vi "ModbusRead.vi"() -> ()   [LabVIEW 2023]
uses:
  <vilib>/NI/Modbus Library/API/Wrapper/Create TCP Master.vi
  <vilib>/NI/Modbus Library/API/Master/Modbus Master.lvclass
  <vilib>/NI/Modbus Library/API/Wrapper/API Main.lvlib
panel:
  in  "register to write":u16
  out "register values":u16[](array[numeric])
  in  "Read":bool
  in  "address":u16
  in  "Write":bool
  in  "stop":bool
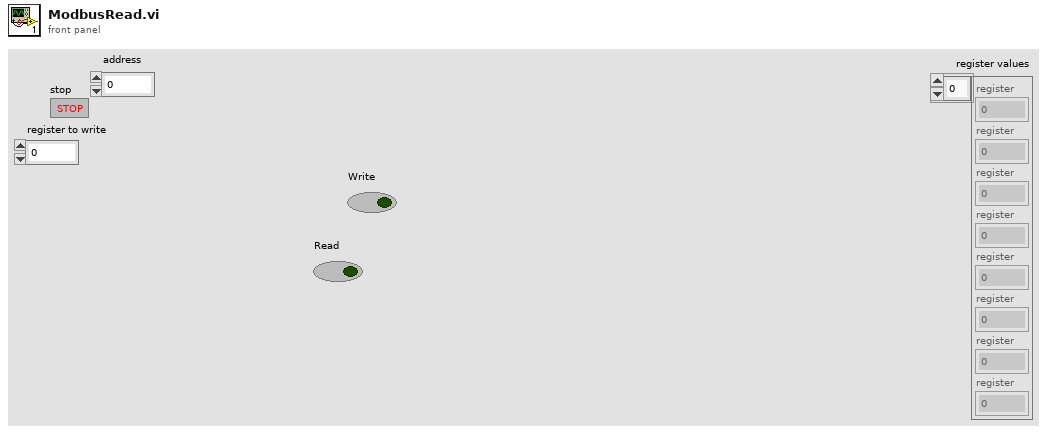
[diagram p1: front panel]
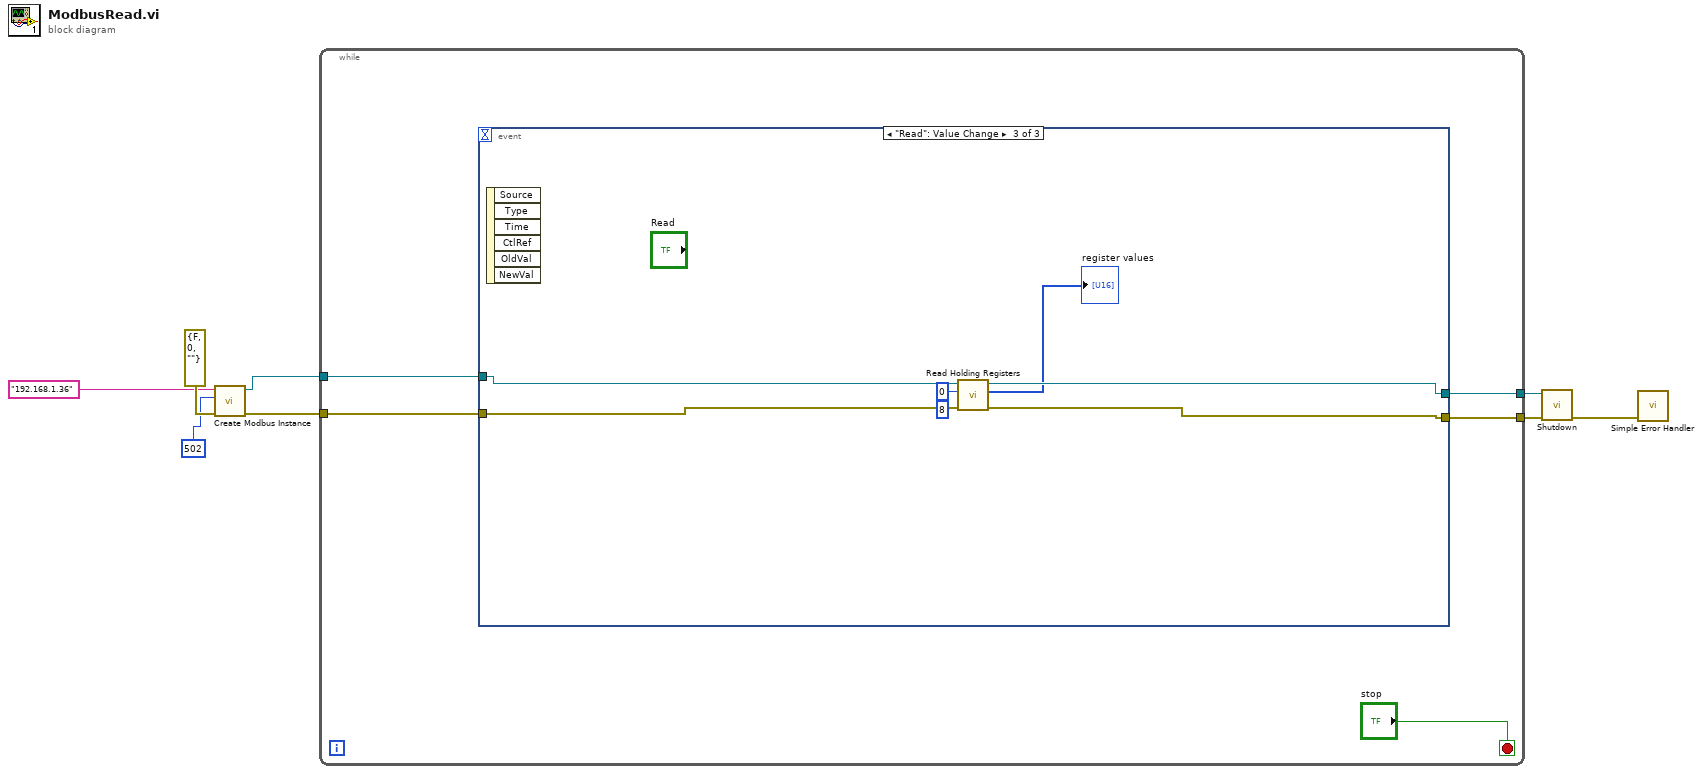
[diagram p0: block diagram]
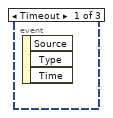
[diagram p2: hidden frame]
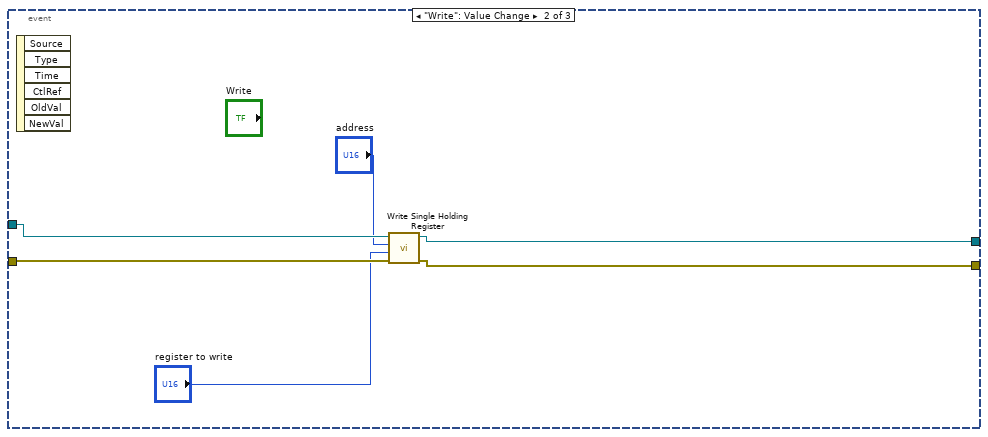
[diagram p3: hidden frame]
diagram:
  n1 = call-poly <vilib>:"Create Modbus Instance.vi"("error in"=errorcluster {"status"=FALSE, "code"=0, "source"=""}, "port (502)"=u16 502, "address"="192.168.1.36") -> ("error out"=w5:errorcluster, "TCP master instance"=w4:refnum<class "Modbus Master.lvclass">)  [unwired: 7 in]
  n2 = while {
    tunnel: w5 -> [w12]
    tunnel: w4 -> [w11]
    tunnel: [w10] -> w3
    tunnel: [w9] -> w2
    stop <- "stop" stop-if-true
    n3 = event shown="[2] \"Read\": Value Change" {
      selector: _ -> [_ _ _]
      dyn-events: _ -> [_ _ _]
      timeout: _ -> [_ _ _]
      tunnel: w12 -> [_ w18 w23]
      tunnel: w11 -> [_ w19 w26]
      tunnel: [_ w17 w24] -> w10
      tunnel: [_ w16 w25] -> w9
      event Timeout {
        n4 = event-data() -> ()  [unwired: 1 in, 3 out]
      }
      event "Write": Value Change {
        n5 = event-data() -> ()  [unwired: 1 in, 6 out]
        n6 = call-dynamic "Write Single Holding Register.vi"("error in"=w18, "register to write"="register to write", "address"="address", "Modbus master in"=w19) -> ("error out"=w17:errorcluster, "Modbus master out"=w16:refnum<class "Modbus Master.lvclass">)  [unwired: 6 in]
      }
      event "Read": Value Change {
        n7 = event-data() -> ()  [unwired: 1 in, 6 out]
        n8 = call-dynamic "Read Holding Registers.vi"("error in"=w23, "number of inputs"=u16 8, "starting address"=u16 0, "Modbus master in"=w26) -> ("error out"=w24:errorcluster, "register values"=→"register values":u16[], "Modbus master out"=w25:refnum<class "Modbus Master.lvclass">)  [unwired: 5 in]
      }
    }
  }
  n9 = call-dynamic "Shutdown.vi"("error in"=w3, "Modbus master in"=w2) -> ("error out"=w1:errorcluster)  [unwired: 9 in]
  n10 = call <vilib>:"Simple Error Handler.vi"("error in (no error)"=w1) -> ()  [unwired: 4 in, 5 out]
